vi "ParseResponse.vi"(8 "error in (no error)":errorcluster, 11 "Response":string) -> (0 "error out":errorcluster, 3 "val":string, 4 "OK":bool, 5 "BD":i32)   [LabVIEW 2018, in "CAEN PSM.lvlib"]
uses:
  <instrlib>/CAEN PSM/CAEN PSM.lvlib
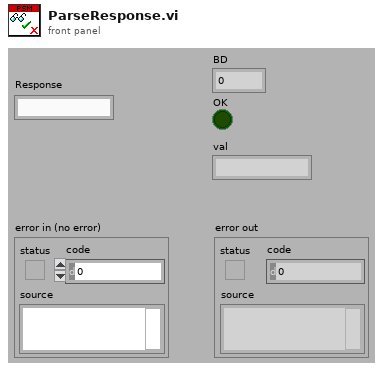
[diagram p1: front panel]
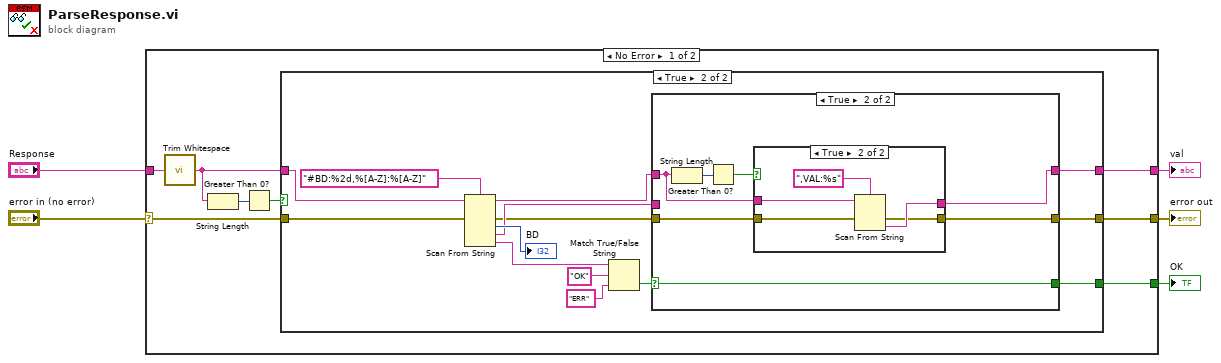
[diagram p0: block diagram]
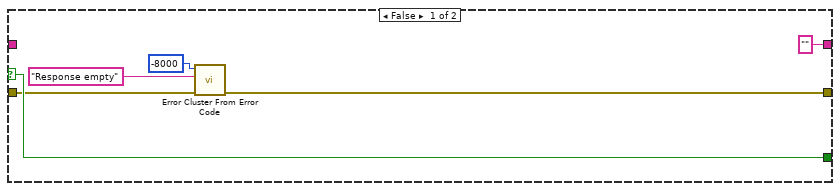
[diagram p2: hidden frame]
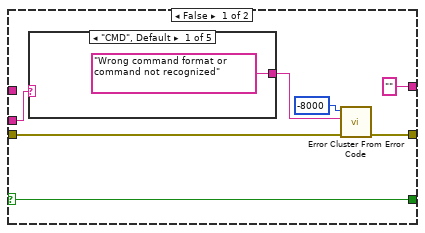
[diagram p3: hidden frame]
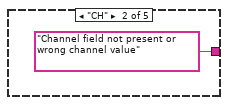
[diagram p4: hidden frame]
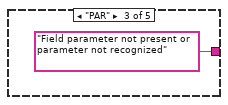
[diagram p5: hidden frame]
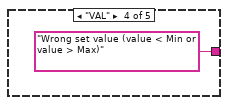
[diagram p6: hidden frame]
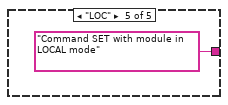
[diagram p7: hidden frame]
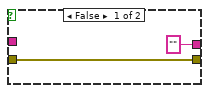
[diagram p8: hidden frame]
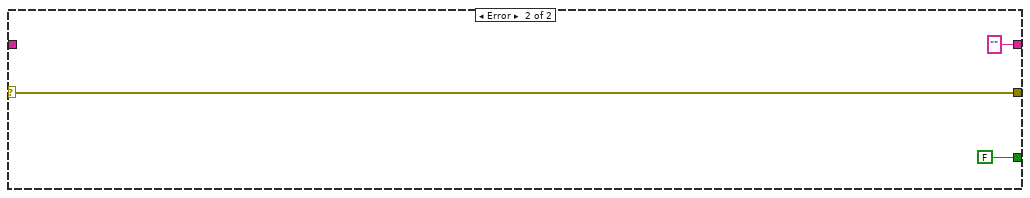
[diagram p9: hidden frame]
diagram:
  n1 = case shown="No Error" "error in (no error)" {
    selector: "error in (no error)" -> [w6 w62]
    tunnel: [w13 ""] -> w5
    tunnel: [w12 w62] -> w4
    tunnel: [w11 FALSE] -> w3
    tunnel: "Response" -> [w8 _]
    frame No Error {
      n2 = call <vilib>:"Trim Whitespace.vi"("string"=w8) -> ("trimmed string"=w7:string)  [unwired: 1 in]
      n3 = String Length(string=w7) -> (length=w10:i32)
      n4 = Greater Than 0?(x=w10) -> (x > 0?=w9:bool)
      n5 = case shown="True" w9 {
        selector: w9 -> [w19 _]
        tunnel: w6 -> [w17 w32]
        tunnel: ["" w27] -> w13
        tunnel: [w18 w26] -> w12
        tunnel: [w19 w25] -> w11
        tunnel: w7 -> [_ w20]
        frame False {
          n6 = call <vilib>:"Error Cluster From Error Code.vi"("error in (no error)"=w17, "error message (\"\")"="Response empty" ("error message (\"\")"), "error code (0)"=-8000) -> ("error out"=w18:errorcluster)  [unwired: 6 in]
        }
        frame True {
          n7 = Scan From String(format string="#BD:%2d,%[A-Z]:%[A-Z]", input string=w20, error in=w32) -> (remaining string=w22:string, error out=w21:errorcluster, output 1=→"BD":i32, output 2=w23:string, output 3=w24:string)  [unwired: 4 in, 1 out]
          n8 = Match True/False String(2:"ERR" ("false string"), 3:"OK" ("true string"), 4:w24) -> (0:w28:bool)  [unwired: 1 out]
          n9 = case shown="True" w28 {
            selector: w28 -> [w34 w49]
            tunnel: w23 -> [w40 _]
            tunnel: w22 -> [_ w48]
            tunnel: ["" w52] -> w27
            tunnel: w21 -> [w37 w51]
            tunnel: [w38 w50] -> w26
            tunnel: [w34 w49] -> w25
            frame False {
              n10 = case shown="\"CMD\", Default" w40 {
                tunnel: ["Wrong command format or command not recognized" "Channel field not present or wrong channel value" "Field parameter not present or parameter not recognized" "Wrong set value (value < Min or value > Max)" "Command SET with module in LOCAL mode"] -> w36
                frame "CMD", Default {
                }
                frame "CH" {
                }
                frame "PAR" {
                }
                frame "VAL" {
                }
                frame "LOC" {
                }
              }
              n11 = call <vilib>:"Error Cluster From Error Code.vi"("error in (no error)"=w37, "error message (\"\")"=w36, "error code (0)"=-8000) -> ("error out"=w38:errorcluster)  [unwired: 6 in]
            }
            frame True {
              n12 = String Length(string=w48) -> (length=w46:i32)
              n13 = Greater Than 0?(x=w46) -> (x > 0?=w47:bool)
              n14 = case shown="True" w47 {
                tunnel: ["" w58] -> w52
                tunnel: w51 -> [w53 w57]
                tunnel: [w53 w56] -> w50
                tunnel: w48 -> [_ w55]
                frame False {
                }
                frame True {
                  n15 = Scan From String(format string=",VAL:%s", input string=w55, error in=w57) -> (error out=w56:errorcluster, output 1=w58:string)  [unwired: 2 in, 2 out]
                }
              }
            }
          }
        }
      }
    }
    frame Error {
    }
  }
  "error out" <- w4
  "val" <- w5
  "OK" <- w3
